vi "LIN Create Session Ref.vi"(0 "Master Frame(3C)":refnum<k21>, 1 "LDF filepath":path, 2 "Slave Frame(3D)":refnum<k21>, 3 "Request Schedule":refnum<k21>, 4 "interface":refnum<k21>, 5 "error in (no error)":errorcluster, 7 "Response Schedule":refnum<k21>) -> (6 "LIN Device":T1={"Master Frame(3C)"="MasterReq\nSPA3414_ConfigurationsCMAGeely_CEMCALYPSOSDB34XX0Cfg_LIN3_190709_", "Slave Frame(3D)"="SlaveResp\nSPA3414_ConfigurationsCMAGeely_CEMCALYPSOSDB34XX0Cfg_LIN3_190709_", "Request Schedule"="CEMLIN3DiagRequestSchedule\nSPA3414_ConfigurationsCMAGeely_CEMCALYPSOSDB34XX0Cfg_LIN3_190709_", "Response Schedule"="CEMLIN3DiagResponseSchedule\nSPA3414_ConfigurationsCMAGeely_CEMCALYPSOSDB34XX0Cfg_LIN3_190709_", "Frame Write SCU"="", "Frame Read SCU"="", "LIN Name"=""}, 8 "错误输出":errorcluster)   [LabVIEW 2018]
uses:
  LIN Device.ctl
  <vilib>/xnet/xnet.llb/XNET Create Session (Frame Output Queued).vi
  <vilib>/xnet/xnet.llb/XNET Create Session (Frame Input Queued).vi
  <resource>/objmgr/xnet.rc
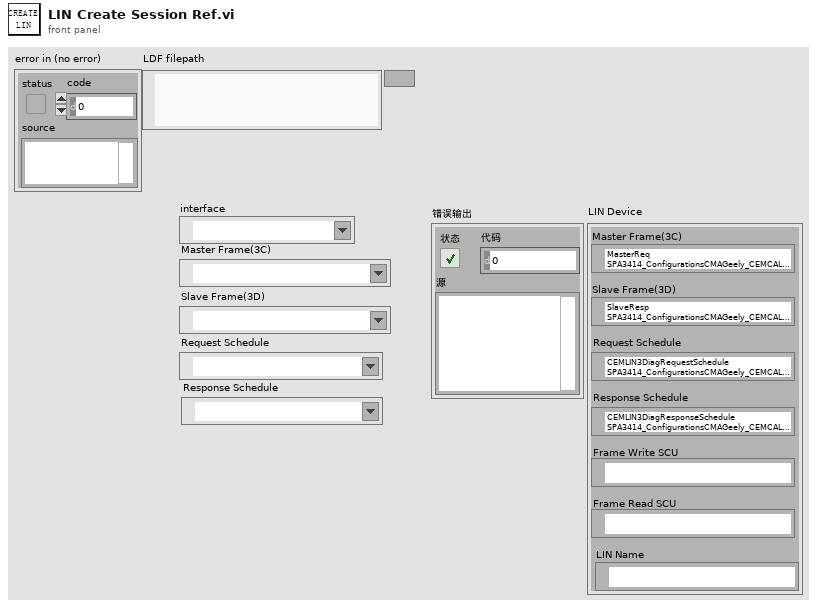
[diagram p1: front panel]
types:
  T1 = typedef "LIN Device.ctl" = cluster{"Master Frame(3C)":refnum<k21>, "Slave Frame(3D)":refnum<k21>, "Request Schedule":refnum<k21>, "Response Schedule":refnum<k21>, "Frame Write SCU":refnum<k21>, "Frame Read SCU":refnum<k21>, "LIN Name":refnum<k21>}
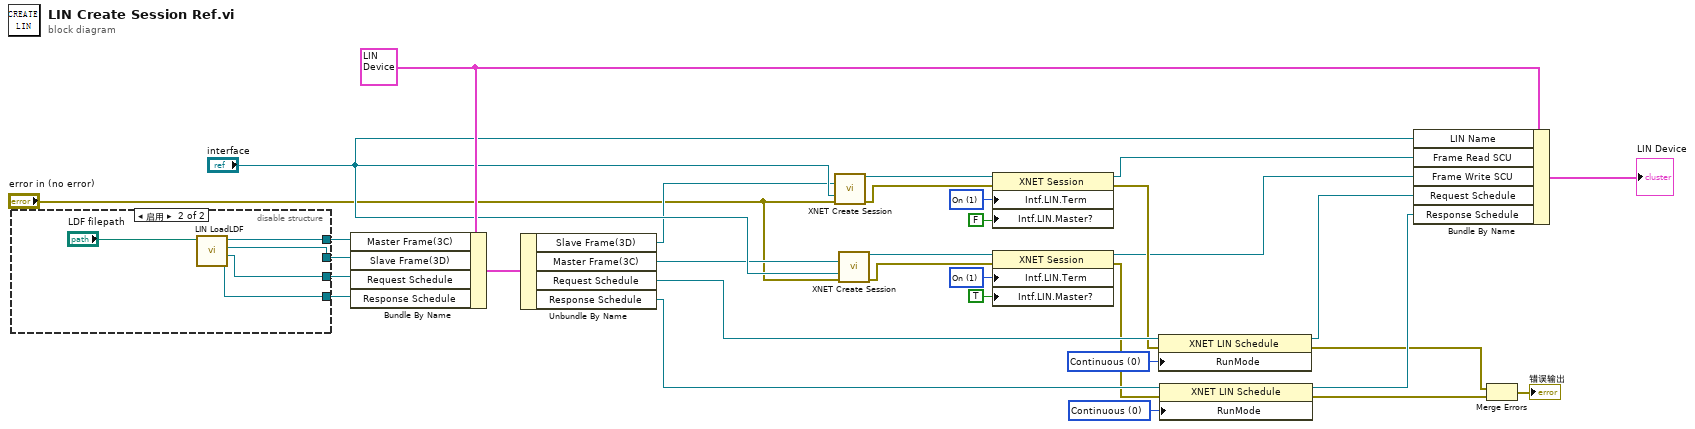
[diagram p0: block diagram]
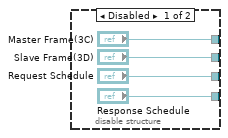
[diagram p2: hidden frame]
diagram:
  w6 = u32 0 items=["Continuous", "Once", "Null"] ("Run Mode")
  w7 = u32 0 items=["Continuous", "Once", "Null"] ("Run Mode")
  w8 = u32 1 items=["Off", "On"] ("Interface:LIN:Termination")
  w9 = u32 1 items=["Off", "On"] ("Interface:LIN:Termination")
  w5 = T1 {"Master Frame(3C)"="MasterReq\nSPA3414_ConfigurationsCMAGeely_CEMCALYPSOSDB34XX0Cfg_LIN3_190709_", "Slave Frame(3D)"="SlaveResp\nSPA3414_ConfigurationsCMAGeely_CEMCALYPSOSDB34XX0Cfg_LIN3_190709_", "Request Schedule"="CEMLIN3DiagRequestSchedule\nSPA3414_ConfigurationsCMAGeely_CEMCALYPSOSDB34XX0Cfg_LIN3_190709_", "Response Schedule"="CEMLIN3DiagResponseSchedule\nSPA3414_ConfigurationsCMAGeely_CEMCALYPSOSDB34XX0Cfg_LIN3_190709_", "Frame Write SCU"="", "Frame Read SCU"="", "LIN Name"=""} ("LIN Device")
  n1 = disable-structure shown="启用" {
    disable-tunnel: ["Master Frame(3C)" w41] -> w32
    disable-tunnel: ["Slave Frame(3D)" w40] -> w31
    disable-tunnel: ["Request Schedule" w39] -> w30
    disable-tunnel: ["Response Schedule" w38] -> w29
    frame Disabled {
    }
    frame Enabled {
      n2 = call "LIN LoadLDF.vi"("filepath"="LDF filepath") -> ("ResponseSchedule"=w38:refnum<k21>, "RequestSchedule"=w39:refnum<k21>, "XNET Frame Slave"=w40:refnum<k21>, "XNET Frame Master"=w41:refnum<k21>)  [unwired: 7 in]
    }
  }
  n3 = Bundle By Name(cluster=w5, "Master Frame(3C)"=w32, "Slave Frame(3D)"=w31, "Request Schedule"=w30, "Response Schedule"=w29) -> (w20:T1)
  n4 = Unbundle By Name(w20) -> ("Slave Frame(3D)"=w3:refnum<k21>, "Master Frame(3C)"=w2:refnum<k21>, "Request Schedule"=w24:refnum<k21>, "Response Schedule"=w23:refnum<k21>)
  n5 = call-poly <vilib>:"XNET Create Session.vi"("frame"=w3, "interface"="interface", "error in (no error)"="error in (no error)") -> ("session out"=w28:refnum<k21>, "error out"=w27:errorcluster)  [unwired: 11 in]
  n6 = call-poly <vilib>:"XNET Create Session.vi"("frame"=w2, "interface"="interface", "error in (no error)"="error in (no error)") -> ("session out"=w26:refnum<k21>, "error out"=w25:errorcluster)  [unwired: 11 in]
  n7 = property class="XNET Session"(reference=w28, error in=w27, "Intf.LIN.Term"=w9, "Intf.LIN.Master?"=FALSE ("Interface:LIN:Master?")) -> (reference out=w19:refnum<k21>, error out=w22:errorcluster)
  n8 = property class="XNET Session"(reference=w26, error in=w25, "Intf.LIN.Term"=w8, "Intf.LIN.Master?"=TRUE ("Interface:LIN:Master?")) -> (reference out=w18:refnum<k21>, error out=w21:errorcluster)
  n9 = property on="属性节点" class="XNET LIN Schedule"(reference=w24, error in=w22, "RunMode"=w7) -> (reference out=w17:refnum<k21>, error out=w15:errorcluster)
  n10 = property on="属性节点" class="XNET LIN Schedule"(reference=w23, error in=w21, "RunMode"=w6) -> (reference out=w16:refnum<k21>, error out=w14:errorcluster)
  n11 = Bundle By Name(cluster=w5, "LIN Name"="interface", "Frame Read SCU"=w19, "Frame Write SCU"=w18, "Request Schedule"=w17, "Response Schedule"=w16) -> (→"LIN Device":T1)
  n12 = Merge Errors(w15, w14) -> (→"错误输出":errorcluster)
